vi "Open Physical Channel Command.vi"(0 "SLSC Interface in":refnum<class "SLSC Interface.lvclass">, 5 "physical channel":refnum<k21>="$DefaultPhysChans", 7 "command in":refnum<k21>, 11 "error in (no error)":errorcluster) -> (4 "SLSC Interface out":refnum<class "SLSC Interface.lvclass">, 8 "command out":refnum<k21>, 15 "error out":errorcluster)   [LabVIEW 2015, in "SLSC Interface.lvclass"]
uses:
  SLSC Interface.lvclass
  slsc type.ctl
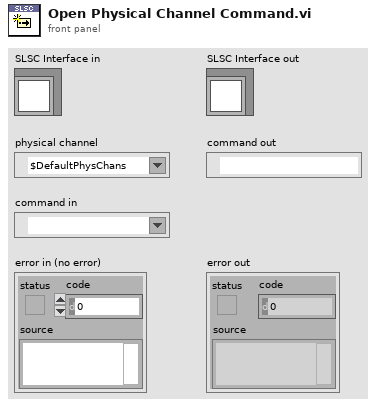
[diagram p1: front panel]
types:
  T1 = typedef "SLSC Interface.lvclass/slsc type.ctl" = enum16{"device", "nvmem", "channel", "none"}
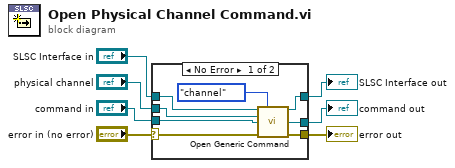
[diagram p0: block diagram]
diagram:
  n1 = case shown="No Error" "error in (no error)" {
    selector: "error in (no error)" -> [w13 w17]
    tunnel: [w12 w17] -> w6
    tunnel: [w14 w16] -> w4
    tunnel: "SLSC Interface in" -> [w15 w16]
    tunnel: "physical channel" -> [w10 _]
    tunnel: [w9 _] -> w2
    tunnel: "command in" -> [w8 _]
    frame No Error {
      n2 = call-dynamic "Open Generic Command.vi"("SLSC Interface in"=w15, "slsc type"=slsc_type."channel", "resource"=w10, "command in"=w8, "error in (no error)"=w13) -> ("SLSC Interface out"=w14:refnum<class "SLSC Interface.lvclass">, "command out"=w9:refnum<k21>, "error out"=w12:errorcluster)  [unwired: 8 in]
    }
    frame Error {
    }
  }
  "error out" <- w6
  "SLSC Interface out" <- w4
  "command out" <- w2
